vi "Wait For Completion.vi"(8 "error in (no error)":errorcluster, 9 "Timeout":u32=5000 caption="ms", 10 "Block on Wait":bool, 11 "Session In":refnum<visa-resource-name>) -> (0 "error out":errorcluster, 3 "Session Out":refnum<visa-resource-name>)   [LabVIEW 2023, in "HAF.lvlib" / "Driver.lvclass"]
doc: "Checks with the Instrument for any running commands, waiting for them to complete.  If Block on Wait is True, then all other processing is blocked until the commands are finished; if False then the processing can continue.\n\nIn either case, the wait will timeout as requested, or after 5 seconds by default."
uses:
  Driver.lvclass
  Driver.lvclass/Driver.ctl
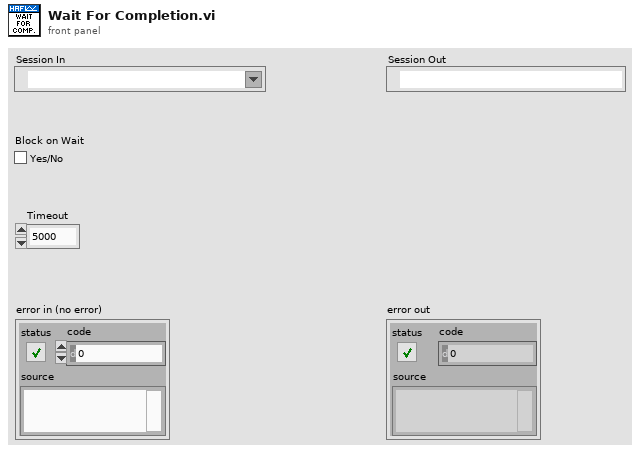
[diagram p1: front panel]
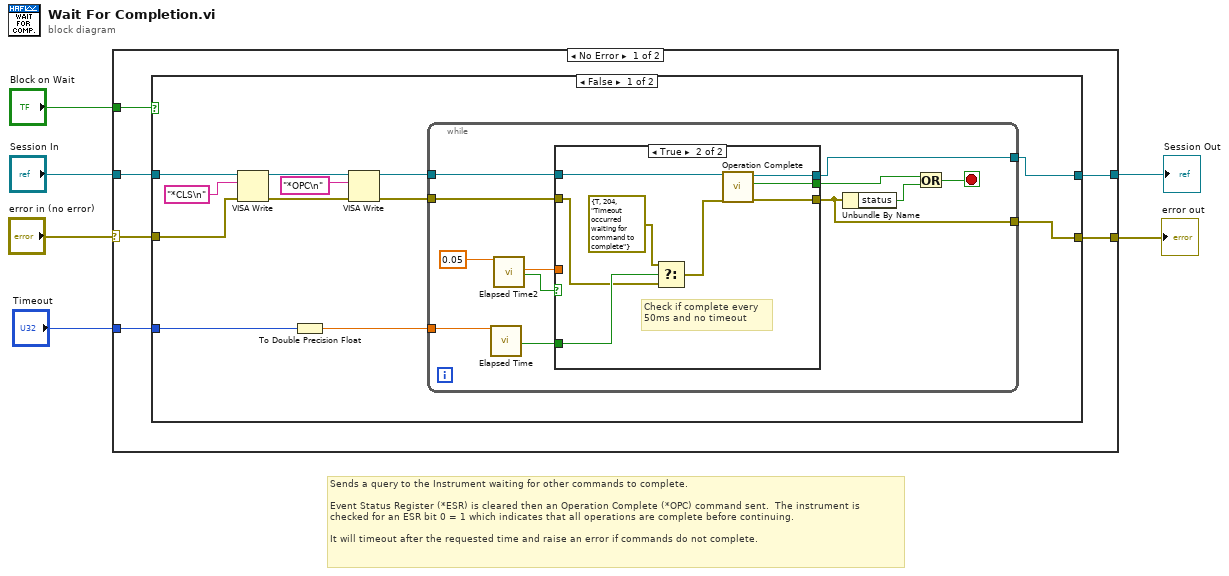
[diagram p0: block diagram]
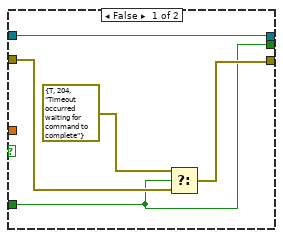
[diagram p2: hidden frame]
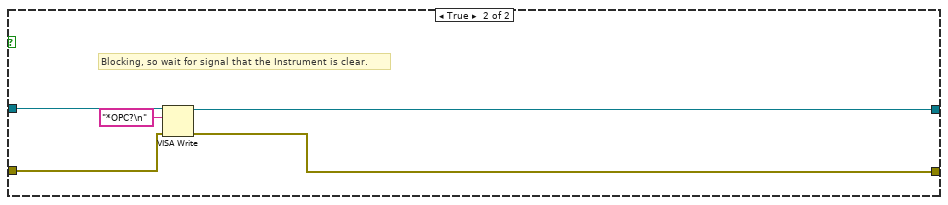
[diagram p3: hidden frame]
diagram:
  # "Sends a query to the Instrument waiting for other commands to complete.\n\nEvent Status Register (*ESR) is cleared then an Operation Complete (*OPC) command sent.  The instrument is\nchecked for an ESR bit 0 = 1 which indicates that all operations are complete before continuing.\n\nIt will timeout after the requested time and raise an error if commands do not complete."
  n1 = case shown="No Error" "error in (no error)" {
    selector: "error in (no error)" -> [w11 w55]
    tunnel: "Session In" -> [w12 w56]
    tunnel: "Timeout" -> [w9 _]
    tunnel: [w8 w56] -> w4
    tunnel: [w7 w55] -> w3
    tunnel: "Block on Wait" -> [w10 _]
    frame No Error {
      n2 = case shown="False" w10 {
        tunnel: w12 -> [w24 w54]
        tunnel: w11 -> [w22 w52]
        tunnel: w9 -> [w16 _]
        tunnel: [w14 w51] -> w8
        tunnel: [w13 w50] -> w7
        frame False {
          n3 = VISA Write(VISA resource name=w24, write buffer="*CLS\n", error in (no error)=w22) -> (VISA resource name out=w21:refnum<visa-resource-name>, error out=w20:errorcluster)  [unwired: 1 out]
          n4 = To Double Precision Float(number=w16) -> (double precision float=w15:dbl)
          n5 = VISA Write(VISA resource name=w21, write buffer="*OPC\n", error in (no error)=w20) -> (VISA resource name out=w18:refnum<visa-resource-name>, error out=w17:errorcluster)  [unwired: 1 out]
          n6 = while {
            tunnel: w18 -> [w35]
            tunnel: w17 -> [w34]
            tunnel: w15 -> [w36]
            tunnel: [w26] -> w14
            tunnel: [w25] -> w13
            stop <- w27 stop-if-true
            n7 = call "Elapsed Time"("Time Target (s)"=w36) -> ("Time has Elapsed"=w30:bool)  [unwired: 11 in, 7 out]
            n8 = call "Elapsed Time2"("Time Target (s)"=0.05) -> ("Elapsed Time (s)"=w32:dbl, "Time has Elapsed"=w33:bool)  [unwired: 11 in, 6 out]
            n9 = case shown="True" w33 {
              tunnel: w35 -> [w41 w46]
              tunnel: w34 -> [w40 w48]
              tunnel: w32 -> [_ _]
              tunnel: w30 -> [w37 w49]
              tunnel: [w41 w44] -> w26
              tunnel: [w37 w43] -> w28
              tunnel: [w38 w42] -> w25
              frame False {
                n10 = Select(t=errorcluster {"status"=TRUE, "code"=204, "source"="Timeout occurred waiting for command to complete"}, s=w37, f=w40) -> (s? t:f=w38:errorcluster)
              }
              frame True {
                # "Check if complete every\n50ms and no timeout"
                n11 = Select(t=errorcluster {"status"=TRUE, "code"=204, "source"="Timeout occurred waiting for command to complete"}, s=w49, f=w48) -> (s? t:f=w45:errorcluster)
                n12 = call "Operation Complete.vi"("error in (no error)"=w45, "Session In"=w46) -> ("error out"=w42:errorcluster, "Operation Complete"=w43:bool, "Session Out"=w44:refnum<visa-resource-name>)  [unwired: 7 in]
              }
            }
            n13 = Unbundle By Name(w25) -> ("status"=w29:bool)
            n14 = Or(x=w28, y=w29) -> (x .or. y?=w27:bool)
          }
        }
        frame True {
          # "Blocking, so wait for signal that the Instrument is clear."
          n15 = VISA Write(VISA resource name=w54, write buffer="*OPC?\n", error in (no error)=w52) -> (VISA resource name out=w51:refnum<visa-resource-name>, error out=w50:errorcluster)  [unwired: 1 out]
        }
      }
    }
    frame Error {
    }
  }
  "Session Out" <- w4
  "error out" <- w3
